vi "Rings on the right.vi"(9 "Separation (angle)":i32, 10 "Revolution (steps)":i32, 11 "Iteration":i32) -> ()   [LabVIEW 2017]
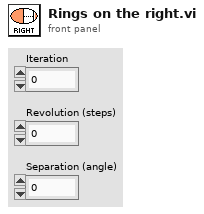
[diagram p1: front panel]
types:
  T1 = enum16{"Full", "Half", "Quarter", "Eighth", "Sixteenth"}
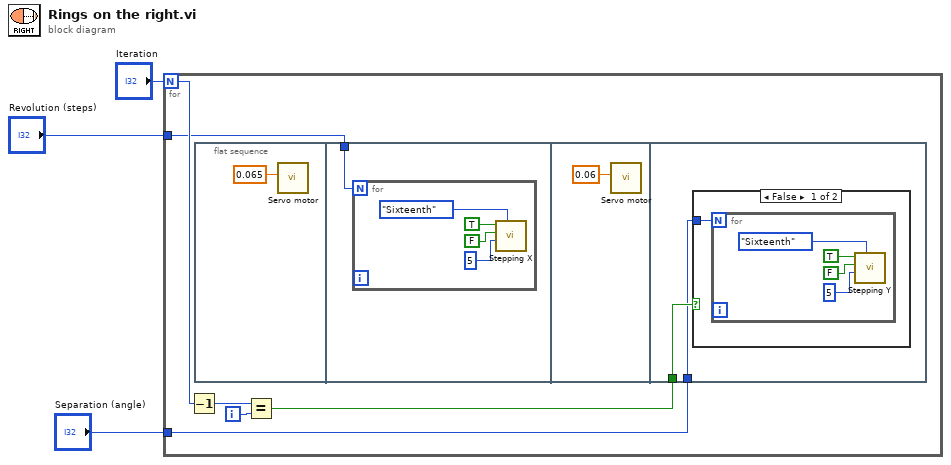
[diagram p0: block diagram]
diagram:
  n1 = for {
    N: "Iteration" -> [w6]
    tunnel: "Revolution (steps)" -> [w5]
    tunnel: "Separation (angle)" -> [w4]
    i -> [w8]
    n2 = Decrement(x=w6) -> (x-1=w9:i32)
    n3 = flat-sequence {
      tunnel: w5 -> [w11]
      tunnel: w7 -> [w18]
      tunnel: w4 -> [w17]
      frame #0 {
        n4 = call "Servo motor.vi"("Duty Cycle"=0.065) -> ()  [unwired: 9 in, 2 out]
      }
      frame #1 {
        n5 = for {
          N: w11 -> [_]
          n6 = call "Stepping X.vi"("Microstep size"=T1."Sixteenth", "Speed"=u32 5, "Direction"=FALSE, "Enable"=TRUE) -> ()  [unwired: 7 in, 1 out]
        }
      }
      frame #2 {
        n7 = call "Servo motor.vi"("Duty Cycle"=0.06) -> ()  [unwired: 9 in, 2 out]
      }
      frame #3 {
        n8 = case shown="False" w18 {
          tunnel: w17 -> [w19 _]
          frame False {
            n9 = for {
              N: w19 -> [_]
              n10 = call "Stepping Y.vi"("Microstep size"=T1."Sixteenth", "Speed"=u32 5, "Direction"=FALSE, "Enable"=TRUE) -> ()  [unwired: 7 in, 1 out]
            }
          }
          frame True {
          }
        }
      }
    }
    n11 = Equal?(x=w9, y=w8) -> (x = y?=w7:bool)
  }
